vi "DatatoGraphNHRRGS.vi"(0 "NHRRGS":refnum<vi>, 7 "Data":variant, 9 "PlotYAxis":u32[](array[numeric]), 11 "error in (no error)":errorcluster) -> (4 "WaveformArray":waveform(dbl)[](array[waveform]), 6 "Incorrect DataType?":bool, 8 "Status Byte Register":T1(array[cluster]), 15 "error out":errorcluster)   [LabVIEW 2018, in "AcPwrModule.lvlib"]
uses:
  AcPwrModule.lvlib
  AcPwrPlugins/NhRegenGridSim/TypeDefs/MeasurementData.ctl
  AcPwrPlugins/NhRegenGridSim/NHRGridSim.lvclass
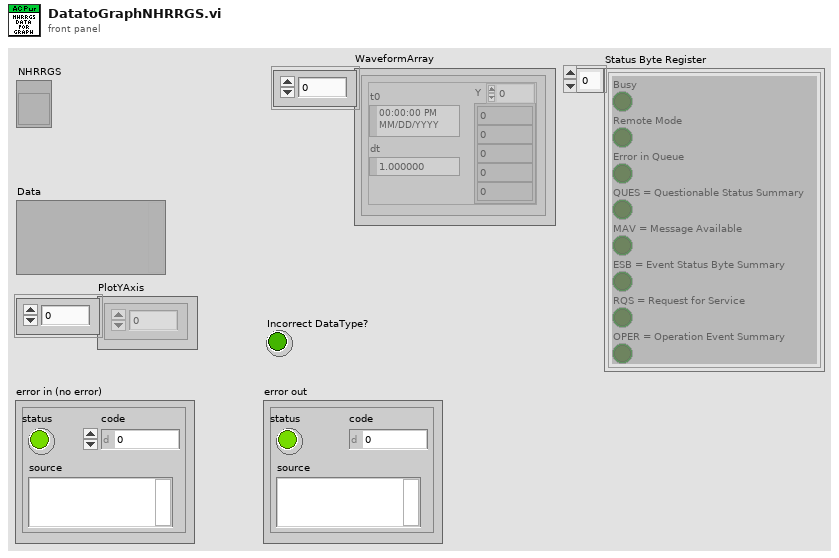
[diagram p1: front panel]
types:
  T1 = cluster{"Busy":bool, "Remote Mode":bool, "Error in Queue":bool, "QUES = Questionable Status Summary":bool, "MAV = Message Available":bool, "ESB = Event Status Byte Summary":bool, "RQS = Request for Service":bool, "OPER = Operation Event Summary":bool}[]
  T2 = typedef "AcPwrPlugins.lvlib/NHRGridSim.lvclass/MeasurementData.ctl" = cluster{"Handle":string, "Waveform":waveform(dbl), "Status Byte Register":cluster{"Busy":bool, "Remote Mode":bool, "Error in Queue":bool, "QUES = Questionable Status Summary":bool, "MAV = Message Available":bool, "ESB = Event Status Byte Summary":bool, "RQS = Request for Service":bool, "OPER = Operation Event Summary":bool}, "Measurement Type ":enum16{"Average Current", "Average Voltage"}}
  T3 = cluster{"Busy":bool, "Remote Mode":bool, "Error in Queue":bool, "QUES = Questionable Status Summary":bool, "MAV = Message Available":bool, "ESB = Event Status Byte Summary":bool, "RQS = Request for Service":bool, "OPER = Operation Event Summary":bool}
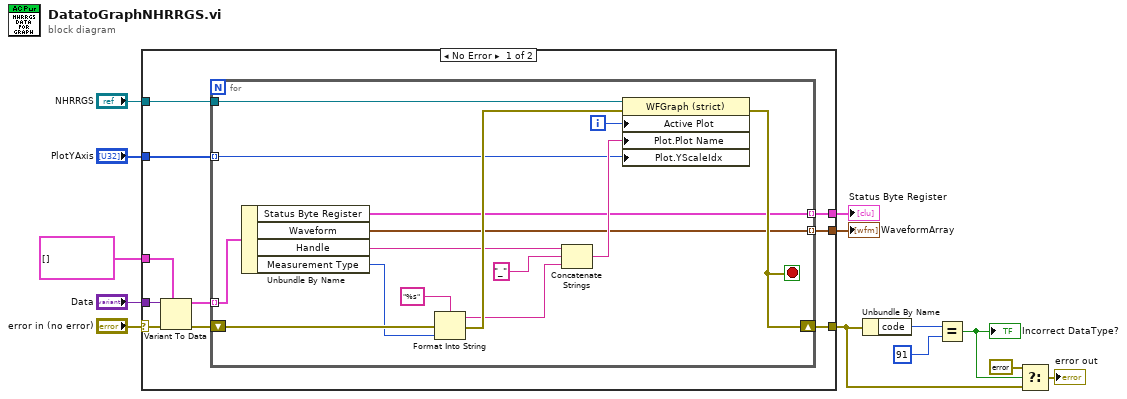
[diagram p0: block diagram]
diagram:
  n1 = case shown="No Error" "error in (no error)" {
    selector: "error in (no error)" -> [w18 w39]
    tunnel: [w23 _] -> w4
    tunnel: "Data" -> [w22 _]
    tunnel: [w21 w39] -> w5
    tunnel: "NHRRGS" -> [w20 _]
    tunnel: "PlotYAxis" -> [w19 _]
    tunnel: T2[] [] ("Array") -> [w16 _]
    tunnel: [w14 _] -> w2
    frame No Error {
      n2 = Variant To Data(error in=w18, type=w16, Variant=w22) -> (data=w15:T2[], error out=w17:errorcluster)
      n3 = for {
        shift-right: [w29] -> w21
        shift-left: w17 -> [w32]
        tunnel: [w27] -> w23 mode=indexing
        tunnel: w20 -> [w31]
        tunnel: w19 -> [w30] mode=indexing
        tunnel: w15 -> [w28] mode=indexing
        tunnel: [w25] -> w14 mode=indexing
        i -> [w38]
        stop <- w29 stop-if-true
        n4 = Unbundle By Name(w28) -> ("Status Byte Register"=w25:T3, "Waveform"=w27:waveform(dbl), "Handle"=w26:string, "Measurement Type"=w24:enum16{"Average Current", "Average Voltage"})
        n5 = Format Into String(format string="%s", error in=w32, w24) -> (resulting string=w35:string, error out=w36:errorcluster)  [unwired: 1 in]
        n6 = Concatenate Strings(w26, "_" ("string"), w35) -> (w34:string)
        n7 = property on="Property Node" class="WFGraph (strict)"(reference=w31, error in=w36, "Active Plot"=w38, "Plot.Plot Name"=w34, "Plot.YScaleIdx"=w30) -> (error out=w29:errorcluster)  [unwired: 1 out]
      }
    }
    frame Error {
    }
  }
  "WaveformArray" <- w4
  "Status Byte Register" <- w2
  n8 = Unbundle By Name(w5) -> ("code"=w10:i32)
  n9 = Equal?(x=w10, y=91) -> (x = y?=w6:bool)
  "Incorrect DataType?" <- w6
  n10 = Select(t=errorcluster {"status"=FALSE, "code"=0, "source"=""} ("error IO"), s=w6, f=w5) -> (s? t:f=→"error out":errorcluster)
